vi "VNA_control.vi"() -> ()   [LabVIEW 2013]
uses:
  <vilib>/Utility/file.llb/Write To Spreadsheet File (DBL).vi
  <vilib>/Utility/file.llb/Write To Spreadsheet File (string).vi
panel:
  in  "Save Graph":bool
  in  "Setup":string="DWU868 Measurement"
  in  "RX antenna":string="MAM-DWU868"
  in  "TX antenna":string="BowTie Vertical"
  in  "Polarization":string="Vertical"
  in  "Save Config":bool
  in  "Config Notes":string="6dB attenuation after Amp\n\n360 turn Antenna in center\nTurntabel pot at 100"
  out "10 deg left":bool
  out "Current Angle":i16=-1
  out "Numeric":i32=2991
  in  "Stop Angle":i16=360
  in  "Start Angle":i16
  in  "Save Current Plot Data":bool
  in  "address":i16=26
  in  "bus":i32
  out "Instrument ID":string="HEWLETT PACKARD,8753ES,US39174843,7.74 \n"
  in  "Number of Points":string="401"
  in  "Output Power":string="0"
  in  "IFBW":string="1000"
  in  "Stop Freq. (MHz)":string="2600"
  out "Forced Sweep Time":string="   4.499999948800000E-01\n"
  out "Forced Start Freq.":string="   1.700000000000000E+09\n"
  out "Forced Stop Freq.":string="   2.600000000000000E+09\n"
  out "Forced IFBW":string="   1.000000000000000E+03\n"
  out "Forced Number of Points":string="   4.010000000000000E+02\n"
  out "Forced  Output Power":string="   0.000000000000000E+00\n"
  in  "Start Freq. (MHz)":string="1700"
  out "Freq. Array":dbl[](array[numeric])=[1700000000.0, 1702250000.0, 1704500000.0, 1706750000.0, 1709000000.0, 1711250000.0, 1713500000.0, 1715750000.0, 1718000000.0, 1720250000.0, 1722500000.0, 1724750000.0, 1727000000.0, 1729250000.0, 1731500000.0, 1733750000.0, 1736000000.0, 1738250000.0, 1740500000.0, 1742750000.0, 1745000000.0, 1747250000.0, 1749500000.0, 1751750000.0, 1754000000.0, 1756250000.0, 1758500000.0, 1760750000.0, 1763000000.0, 1765250000.0, 1767500000.0, 1769750000.0, 1772000000.0, 1774250000.0, 1776500000.0, 1778750000.0, 1781000000.0, 1783250000.0, 1785500000.0, 1787750000.0, 1790000000.0, 1792250000.0, 1794500000.0, 1796750000.0, 1799000000.0, 1801250000.0, 1803500000.0, 1805750000.0, 1808000000.0, 1810250000.0, 1812500000.0, 1814750000.0, 1817000000.0, 1819250000.0, 1821500000.0, 1823750000.0, 1826000000.0, 1828250000.0, 1830500000.0, 1832750000.0, 1835000000.0, 1837250000.0, 1839500000.0, 1841750000.0, 1844000000.0, 1846250000.0, 1848500000.0, 1850750000.0, 1853000000.0, 1855250000.0, 1857500000.0, 1859750000.0, 1862000000.0, 1864250000.0, 1866500000.0, 1868750000.0, 1871000000.0, 1873250000.0, 1875500000.0, 1877750000.0, 1880000000.0, 1882250000.0, 1884500000.0, 1886750000.0, 1889000000.0, 1891250000.0, 1893500000.0, 1895750000.0, 1898000000.0, 1900250000.0, 1902500000.0, 1904750000.0, 1907000000.0, 1909250000.0, 1911500000.0, 1913750000.0, 1916000000.0, 1918250000.0, 1920500000.0, 1922750000.0, 1925000000.0, 1927250000.0, 1929500000.0, 1931750000.0, 1934000000.0, 1936250000.0, 1938500000.0, 1940750000.0, 1943000000.0, 1945250000.0, 1947500000.0, 1949750000.0, 1952000000.0, 1954250000.0, 1956500000.0, 1958750000.0, 1961000000.0, 1963250000.0, 1965500000.0, 1967750000.0, 1970000000.0, 1972250000.0, 1974500000.0, 1976750000.0, 1979000000.0, 1981250000.0, 1983500000.0, 1985750000.0, 1988000000.0, 1990250000.0, 1992500000.0, 1994750000.0, 1997000000.0, 1999250000.0, 2001500000.0, 2003750000.0, 2006000000.0, 2008250000.0, 2010500000.0, 2012750000.0, 2015000000.0, 2017250000.0, 2019500000.0, 2021750000.0, 2024000000.0, 2026250000.0, 2028500000.0, 2030750000.0, 2033000000.0, 2035250000.0, 2037500000.0, 2039750000.0, 2042000000.0, 2044250000.0, 2046500000.0, 2048750000.0, 2051000000.0, 2053250000.0, 2055500000.0, 2057750000.0, 2060000000.0, 2062250000.0, 2064500000.0, 2066750000.0, 2069000000.0, 2071250000.0, 2073500000.0, 2075750000.0, 2078000000.0, 2080250000.0, 2082500000.0, 2084750000.0, 2087000000.0, 2089250000.0, 2091500000.0, 2093750000.0, 2096000000.0, 2098250000.0, 2100500000.0, 2102750000.0, 2105000000.0, 2107250000.0, 2109500000.0, 2111750000.0, 2114000000.0, 2116250000.0, 2118500000.0, 2120750000.0, 2123000000.0, 2125250000.0, 2127500000.0, 2129750000.0, 2132000000.0, 2134250000.0, 2136500000.0, 2138750000.0, 2141000000.0, 2143250000.0, 2145500000.0, 2147750000.0, 2150000000.0, 2152250000.0, 2154500000.0, 2156750000.0, 2159000000.0, 2161250000.0, 2163500000.0, 2165750000.0, 2168000000.0, 2170250000.0, 2172500000.0, 2174750000.0, 2177000000.0, 2179250000.0, 2181500000.0, 2183750000.0, 2186000000.0, 2188250000.0, 2190500000.0, 2192750000.0, 2195000000.0, 2197250000.0, 2199500000.0, 2201750000.0, 2204000000.0, 2206250000.0, 2208500000.0, 2210750000.0, 2213000000.0, 2215250000.0, 2217500000.0, 2219750000.0, 2222000000.0, 2224250000.0, 2226500000.0, 2228750000.0, 2231000000.0, 2233250000.0, 2235500000.0, 2237750000.0, 2240000000.0, 2242250000.0, 2244500000.0, 2246750000.0, 2249000000.0, 2251250000.0, 2253500000.0, 2255750000.0, 2258000000.0, 2260250000.0, 2262500000.0, 2264750000.0, 2267000000.0, 2269250000.0, 2271500000.0, 2273750000.0, 2276000000.0, 2278250000.0, 2280500000.0, 2282750000.0, 2285000000.0, 2287250000.0, 2289500000.0, 2291750000.0, 2294000000.0, 2296250000.0, 2298500000.0, 2300750000.0, 2303000000.0, 2305250000.0, 2307500000.0, 2309750000.0, 2312000000.0, 2314250000.0, 2316500000.0, 2318750000.0, 2321000000.0, 2323250000.0, 2325500000.0, 2327750000.0, 2330000000.0, 2332250000.0, 2334500000.0, 2336750000.0, 2339000000.0, 2341250000.0, 2343500000.0, 2345750000.0, 2348000000.0, 2350250000.0, 2352500000.0, 2354750000.0, 2357000000.0, 2359250000.0, 2361500000.0, 2363750000.0, 2366000000.0, 2368250000.0, 2370500000.0, 2372750000.0, 2375000000.0, 2377250000.0, 2379500000.0, 2381750000.0, 2384000000.0, 2386250000.0, 2388500000.0, 2390750000.0, 2393000000.0, 2395250000.0, 2397500000.0, 2399750000.0, 2402000000.0, 2404250000.0, 2406500000.0, 2408750000.0, 2411000000.0, 2413250000.0, 2415500000.0, 2417750000.0, 2420000000.0, 2422250000.0, 2424500000.0, 2426750000.0, 2429000000.0, 2431250000.0, 2433500000.0, 2435750000.0, 2438000000.0, 2440250000.0, 2442500000.0, 2444750000.0, 2447000000.0, 2449250000.0, 2451500000.0, 2453750000.0, 2456000000.0, 2458250000.0, 2460500000.0, 2462750000.0, 2465000000.0, 2467250000.0, 2469500000.0, 2471750000.0, 2474000000.0, 2476250000.0, 2478500000.0, 2480750000.0, 2483000000.0, 2485250000.0, 2487500000.0, 2489750000.0, 2492000000.0, 2494250000.0, 2496500000.0, 2498750000.0, 2501000000.0, 2503250000.0, 2505500000.0, 2507750000.0, 2510000000.0, 2512250000.0, 2514500000.0, 2516750000.0, 2519000000.0, 2521250000.0, 2523500000.0, 2525750000.0, 2528000000.0, 2530250000.0, 2532500000.0, 2534750000.0, 2537000000.0, 2539250000.0, 2541500000.0, 2543750000.0, 2546000000.0, 2548250000.0, 2550500000.0, 2552750000.0, 2555000000.0, 2557250000.0, 2559500000.0, 2561750000.0, 2564000000.0, 2566250000.0, 2568500000.0, 2570750000.0, 2573000000.0, 2575250000.0, 2577500000.0, 2579750000.0, 2582000000.0, 2584250000.0, 2586500000.0, 2588750000.0, 2591000000.0, 2593250000.0, 2595500000.0, 2597750000.0, 2600000000.0]
  in  "Initiate VNA":bool
  in  "Start Turntabel":bool
  out "output array":dbl[](array[numeric])=[-46.14952865404781, -46.232691273557066, -46.2430751503902, -47.25114271797669, -48.120198903692916, -48.730730027922824, -49.09122541047449, -48.90673988745354, -48.544485930725855, -47.554193224998116, -46.87496927167575, -47.323185912630805, -47.33524101209766, -47.700566092891414, -47.92224440903191, -48.31440966542858, -48.44676619037045, -48.369140911799356, -47.9319832767418, -47.79400417552629, -47.695877874655494, -47.27824599163412, -47.543545591805994, -47.85140868427288, -48.01611296880547, -48.53975692801747, -49.98407852530598, -50.26084058142029, -51.97096924166111, -52.47408937498201, -52.98432913841936, -52.98251865389443, -53.182245088383866, -53.73887271810353, -54.03381513974967, -54.53405597057487, -55.14036079577603, -55.09964293760475, -54.37403089032421, -54.509993323127986, -54.132221772847686, -53.93974466854097, -53.872323842183405, -54.5572260055185, -55.082787936170085, -54.76082910636844, -55.36994774177763, -55.04309671548235, -55.05711705014066, -54.743857051015546, -54.95419359130922, -55.453231036245526, -56.620040992534314, -56.933180240449126, -57.98254486940575, -58.47116123008044, -57.63144943704836, -56.354612757402826, -56.33945467985886, -55.55041492411028, -55.13498792296701, -54.98928915550141, -53.54147323007345, -53.0866987847333, -51.49720736907496, -50.65872377331299, -49.429444691265175, -49.00066533585979, -49.18236382208785, -48.7346651816435, -48.6428733454471, -49.0369511760136, -49.647405916877204, -49.91495131123127, -50.73332378781956, -51.146640766658365, -53.274167053780715, -53.07556548774521, -54.967399293132374, -54.91558848425554, -54.981529686395916, -53.81281146841167, -52.721668856936496, -52.29174907211479, -51.30755297551491, -51.555344613413695, -51.49437195127626, -50.859642725917915, -50.47279848060345, -50.16547905504841, -49.515991937660516, -48.996309364354886, -48.5516751819824, -49.024107657150886, -49.91174729634915, -50.07206023503437, -50.354983564457726, -50.392253363720755, -50.47806698290641, -51.51467197522007, -51.351231626270355, -51.69316044997287, -53.26430703058692, -54.35675089190596, -54.85802150691952, -54.704993318181884, -55.76726541464235, -54.59961731237464, -53.30318902070684, -52.94609349489569, -52.022734676258466, -52.11828429214016, -51.638575770160706, -51.01379988123214, -50.81589628452204, -50.87648726039296, -50.574567626726726, -50.64041926852853, -51.23049863941315, -52.77518876786951, -54.565252786618956, -55.67713448969707, -54.97657805901591, -55.08819292455469, -53.636596755806, -52.06216902185375, -51.753902007901964, -51.362001769216164, -51.22852523767171, -50.859218499788064, -51.50091639754157, -52.16908806766697, -52.20245674039589, -52.78518708052982, -52.48479007561359, -52.32892136658103, -52.26852911390827, -52.13380162088395, -51.77905530163895, -52.735823457055815, -53.81481636754703, -54.75341742214041, -54.940658392596305, -56.054572522496755, -58.47243572834671, -57.76124622271905, -57.058175267930274, -56.269775356868635, -55.045786149128375, -53.446627798069, -52.86588443898755, -53.08744436022421, -53.11735575591441, -53.765960092523606, -54.04943344923838, -53.86246333075452, -53.63391540269025, -52.562326184283066, -52.18242551834151, -51.662691717319504, -52.048603771022385, -51.96139467528154, -52.349486330100284, -53.071788933659725, -53.915943306995786, -55.505890401255925, -56.576757954112225, -57.4142046921861, -60.01099137822906, -58.18265447419201, -58.46272582985546, -56.72814383384765, -56.138856824351464, -54.92303353601231, -54.13069037615369, -54.041884744102695, -53.52403819998679, -52.75135112760272, -52.664887440409785, -51.46976083524018, -51.585128029137564, -51.31789520890483, -50.968888605370694, -50.84010994573585, -51.375048830498145, -51.4022248032098, -51.79429768890644, -52.64804024181253, -53.95089200145986, -55.64999686317979, -56.527693517294004, -57.93929882997876, -58.18334879548402, -56.74120095178944, -56.32073895503707, -55.095781520608696, -54.640016588348104, -54.16375042634547, -53.54090662420656, -53.155620894520524, -52.89394954756738, -52.14525498371656, -52.14636786851274, -52.25143622782487, -52.823523428578156, -54.17398555442098, -54.36688985412034, -54.34227843986237, -54.58314609059877, -54.57723755565346, -54.105672986039856, -54.889370038295866, -55.98966342846481, -57.24096049907829, -59.98627732389639, -58.50017548457405, -58.501426766481714, -56.23661821314542, -54.95043675718922, -54.127780510113, -53.450576979909385, -53.63090794550815, -53.928380762141984, -54.13683658276507, -54.540962001289415, -54.86955512548106, -55.34394924932282, -55.15981874534231, -55.28640089518934, -55.46842364266997, -55.81223725249389, -56.395570583459175, -56.29175492961587, -56.83404549292931, -57.8393031277243, -57.64316593133805, -57.29374553728293, -57.00104583682321, -57.57344727121647, -58.09325416171514, -57.57483582826591, -55.78214269066137, -55.261525588080794, -54.02783172166294, -53.57537740207282, -53.52052550346449, -53.68735889131014, -55.18092983656392, -56.34549876165538, -55.918397497849746, -55.35119850754077, -55.94772721336473, -55.82941229807342, -55.20278579555211, -54.948624944647776, -55.96472293595988, -56.93216605743473, -56.62091714768949, -56.344134807314, -56.87589189638767, -58.07588784043862, -56.61746447511564, -57.37793393626014, -56.544796647017954, -56.84017188827894, -55.6548966978255, -54.893537730518986, -53.959397461583514, -55.03887939804265, -54.965845039381584, -54.31395807000967, -54.358759341780285, -55.33356078933967, -56.225359077155275, -55.65103376805243, -55.26348670787047, -55.467908232117686, -55.16848650302911, -54.88731484218719, -54.9758391979146, -55.64412397666068, -56.96934756557026, -57.65955600340944, -55.916224294186776, -55.612167236283405, -55.96308576364933, -56.05231864509027, -55.25347599171945, -55.304583268840524, -55.69757297967533, -56.195809454262246, -54.82790811670832, -54.31342240066522, -54.6145369456925, -54.4531761464751, -53.96187197225166, -53.78090109665749, -53.85330013355278, -54.31466736083655, -54.5671580183431, -54.40724045187317, -55.490000620727315, -56.18920098061764, -57.25904466242302, -58.243628500935955, -58.79003501603385, -60.14505058874654, -60.14278073191541, -60.07809070689417, -57.809595741609165, -58.25229962043673, -58.33514185743652, -58.27537699051207, -57.982458817507876, -57.32506348305857, -56.66224565603442, -55.51869934148086, -54.691925020045645, -54.10692375027259, -54.900046526270444, -54.933692151675906, -56.019032428599985, -55.34456759853007, -55.953658267597184, -56.3791344707824, -56.26438578443476, -56.93526534183916, -57.33423251579217, -58.07822806088768, -58.76243251365143, -58.67133015427089, -58.28982113165295, -58.95225990994228, -58.67126209522736, -57.89987614108138, -57.72620629786993, -57.62425975451958, -56.97306879778283, -57.70848962384082, -57.357219867042076, -57.42349439048927, -57.64482666750731, -58.34784235225299, -57.311726932236496, -57.09929950493894, -57.04169634219369, -57.9138740414414, -57.726322625896415, -57.43839965210705, -57.30879814697985, -57.40503608346495, -56.91037950988086, -57.31970259346343, -58.5831639851512, -59.57149175879184, -60.71303717626585, -61.48630455672968, -61.31227523849908, -61.539120672976686, -60.982442738400195, -60.83008160295606, -60.3810650516995, -60.11182688482912, -60.14622384911674, -59.536412725623045, -58.466165432555556, -58.211492553458406, -57.70695649674601, -56.87189462723518, -56.347512153121706, -56.03399358565113, -56.42318400860642, -57.28869218804995, -58.22846603399611, -58.63279363791775, -58.59667261259264, -59.005226463047904, -58.815012450001504, -58.33561529066227, -58.02667764914552, -58.33733261314406, -58.62425246039699, -58.040265154895366, -56.91046547462501, -57.706983087948785, -59.010485928120886, -58.97101422590738, -59.0853283186, -59.39769414728251, -60.25211579991711, -59.7957969175217, -59.46973747494233, -58.84867051731946, -58.732266964976205, -58.63718591494741, -58.359292232606315, -58.15315438077847, -58.86195256988518, -59.5661822007773, -60.74784745212166, -60.516354440305406]
  in  "Capture Data":bool
  in  "stop":bool
  out "XY Graph":cluster{"Freq. Array":dbl[], dbl[]}(graph)
  in  "Serial Port":refnum<visa-resource-name>="ASRL4::INSTR"
  out "DCD":bool
  # "SMP VNA: 26"
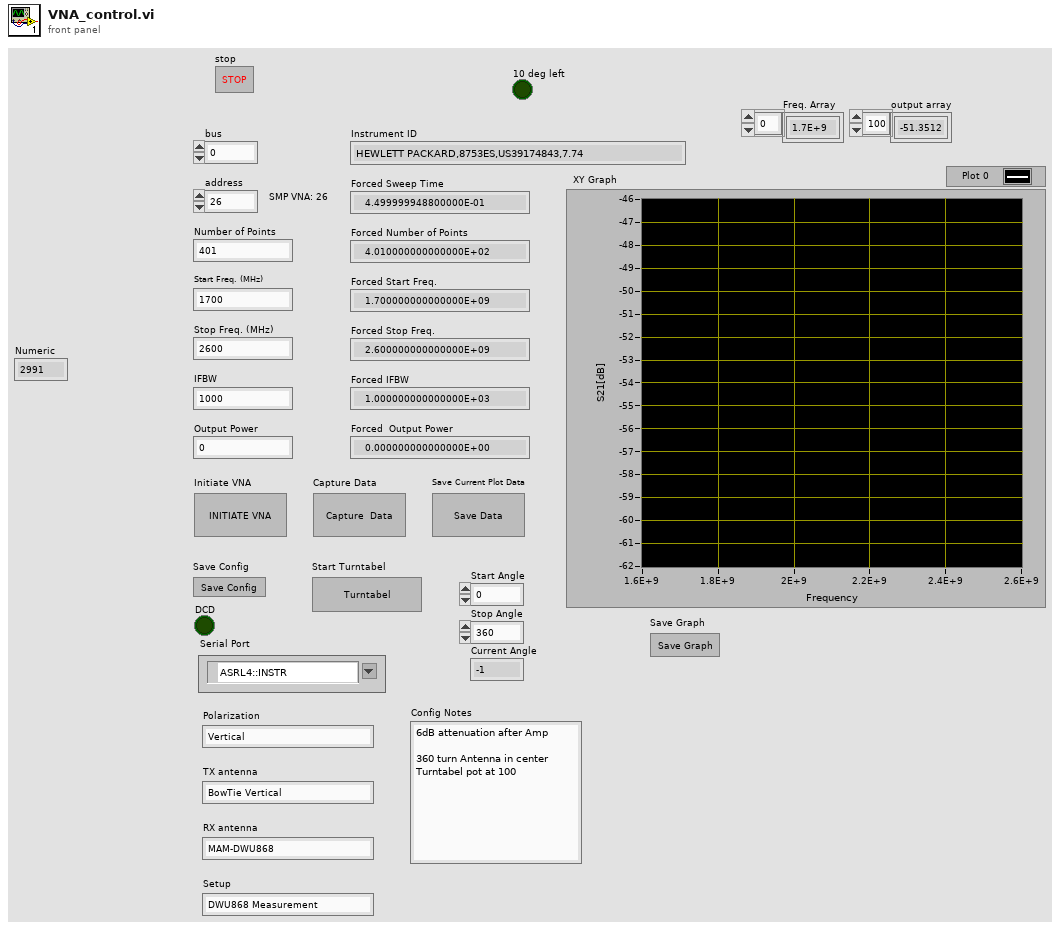
[diagram p1: front panel]
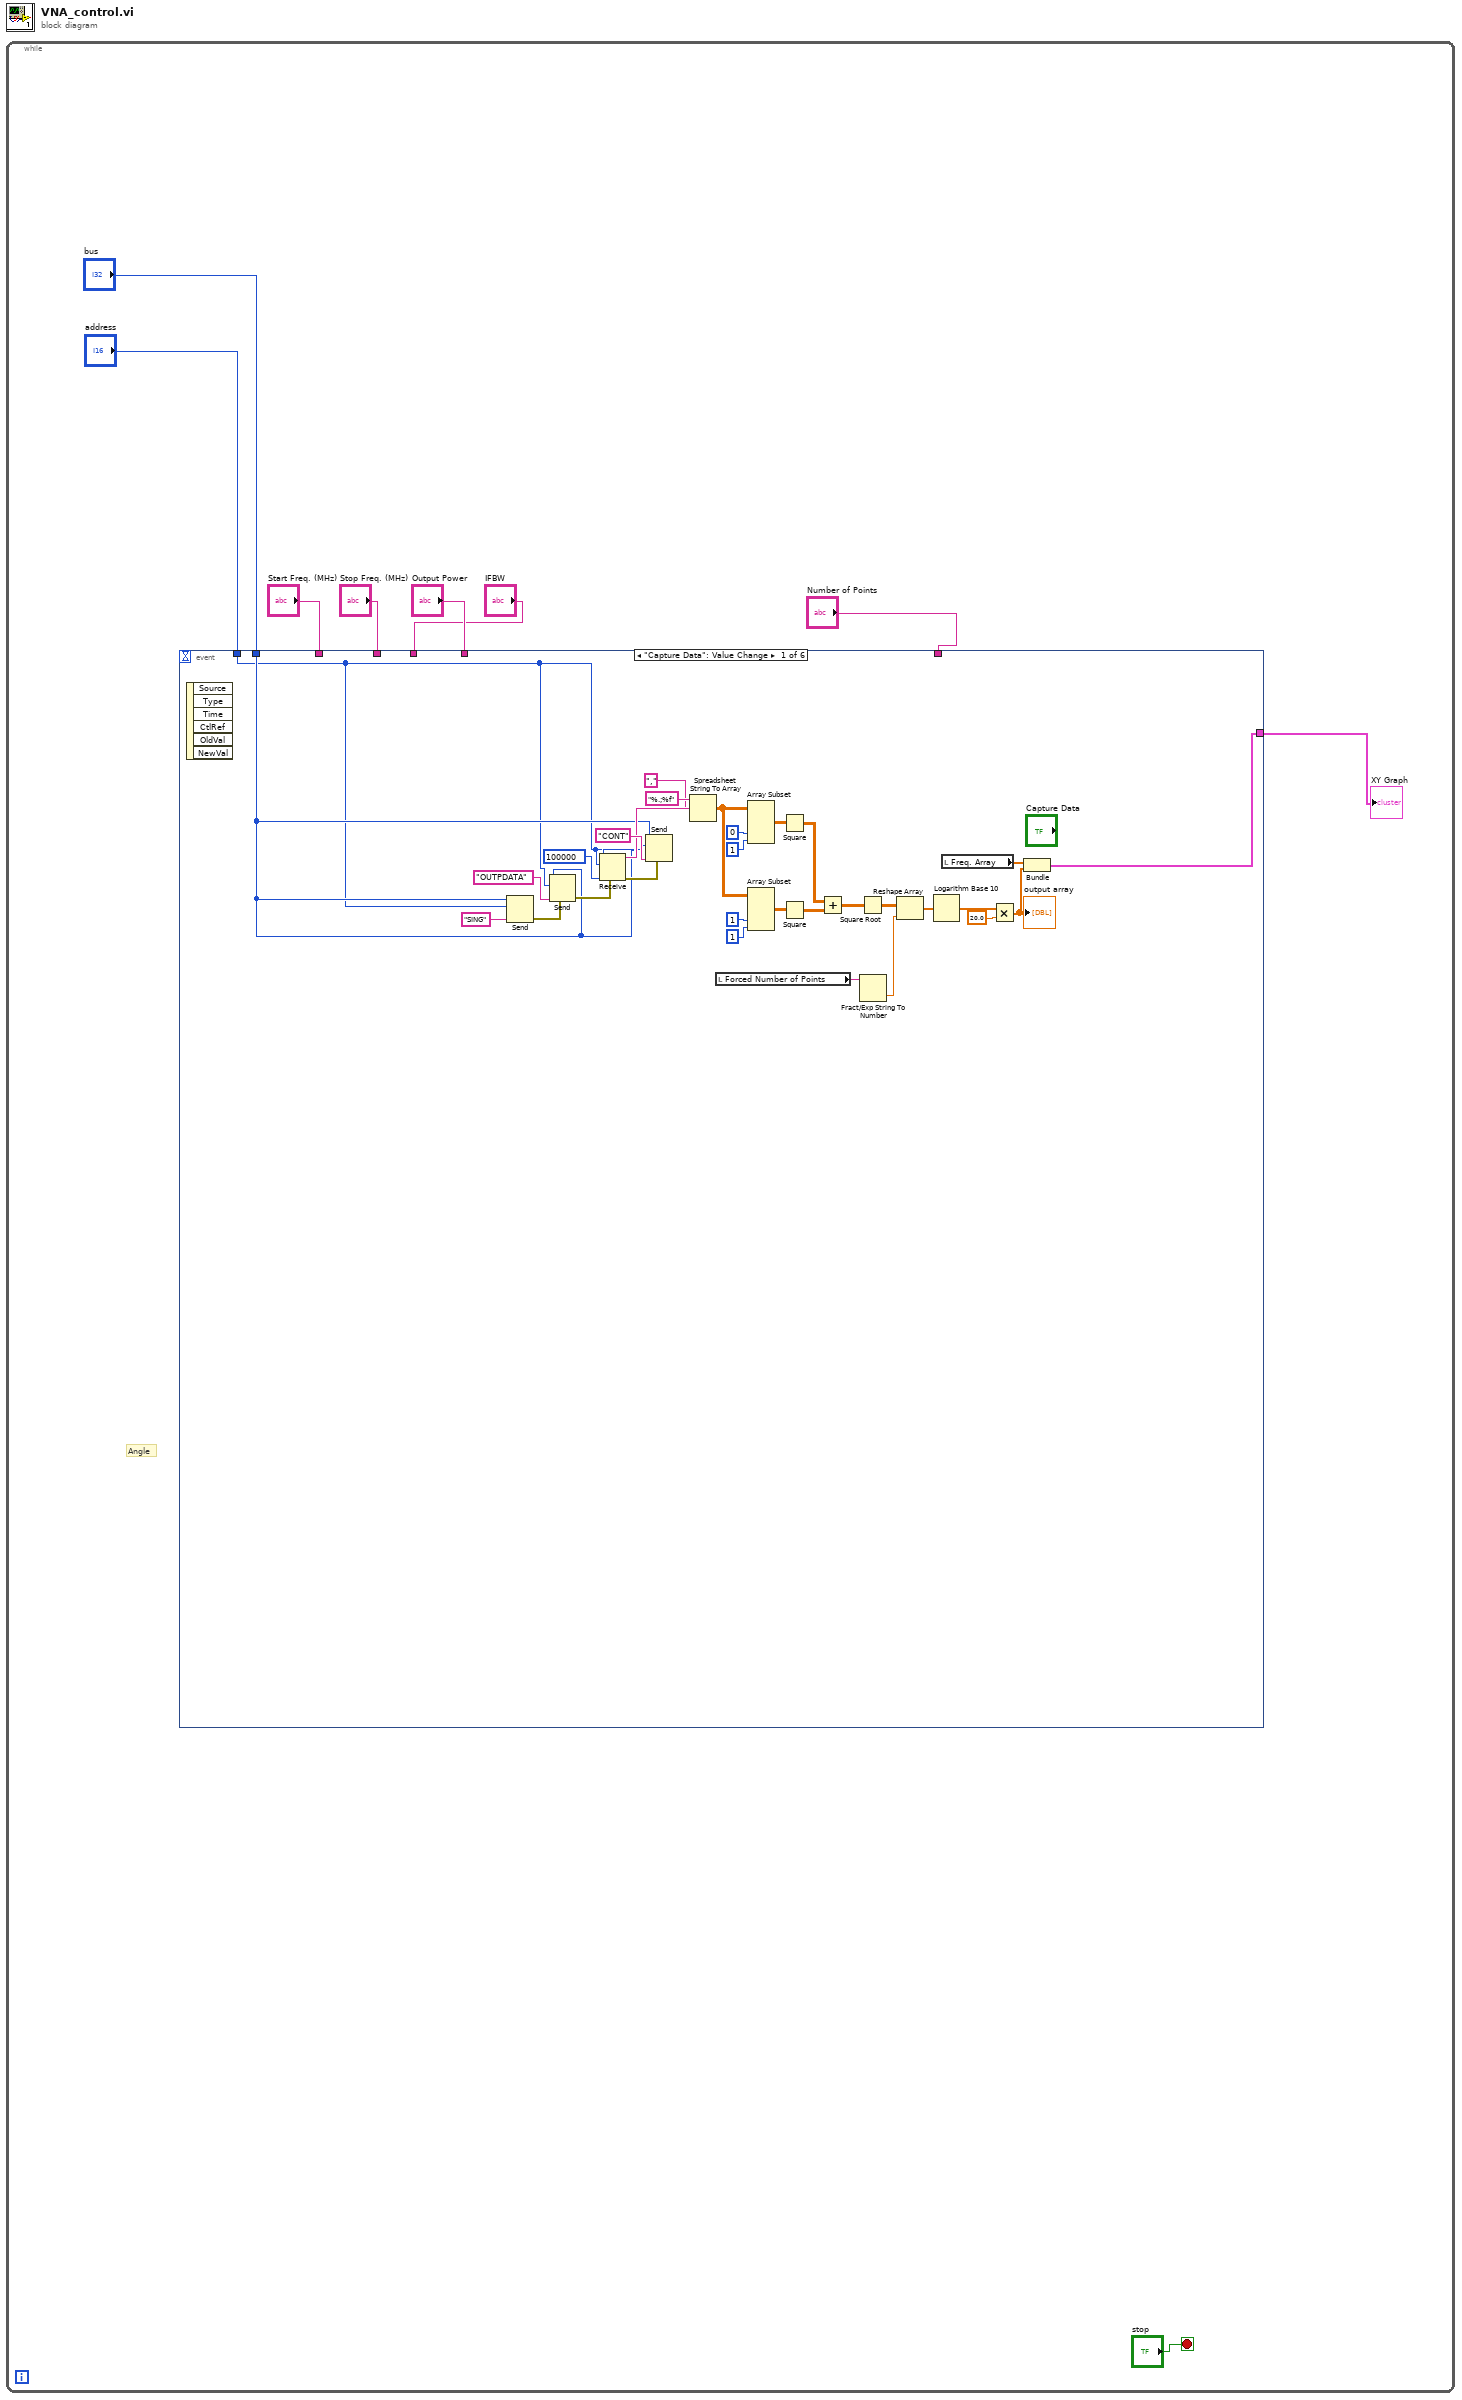
[diagram p0: block diagram]
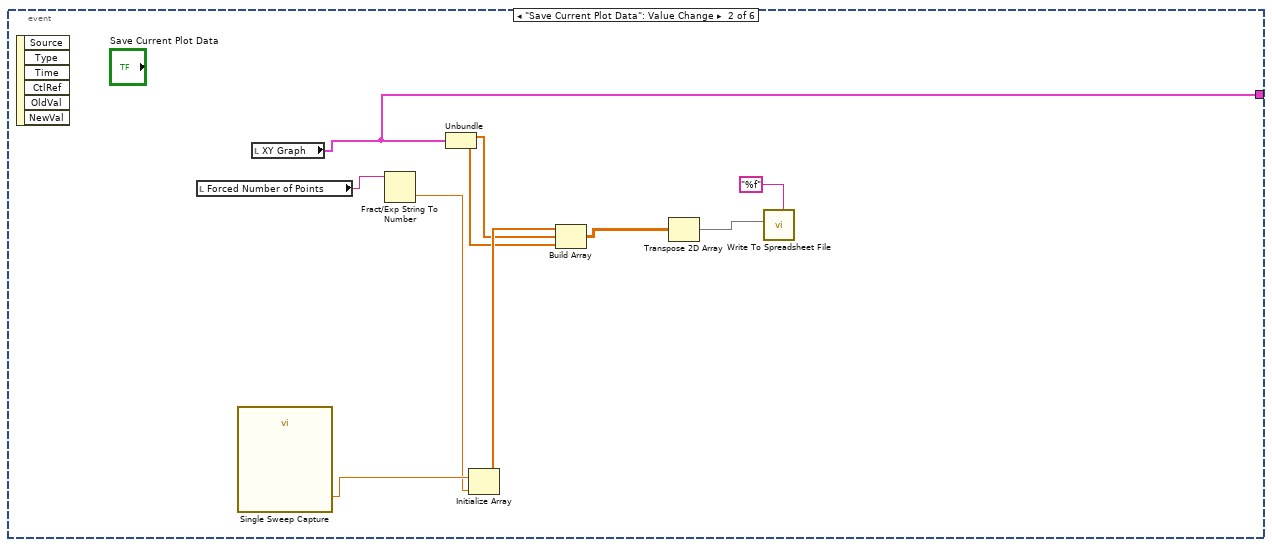
[diagram p2: hidden frame]
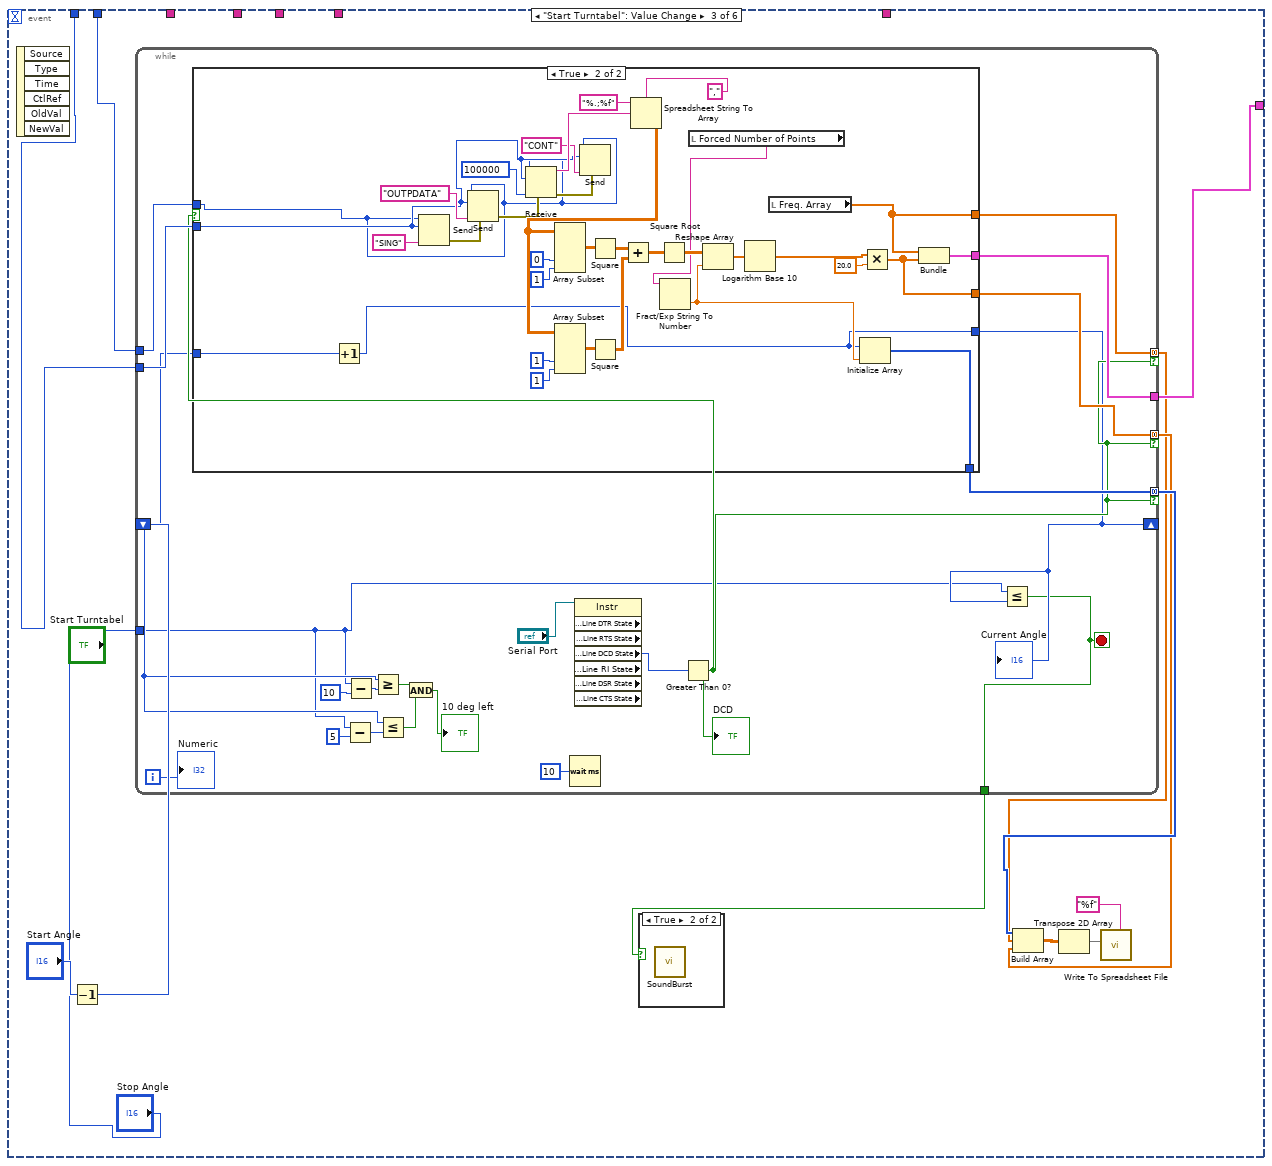
[diagram p3: hidden frame]
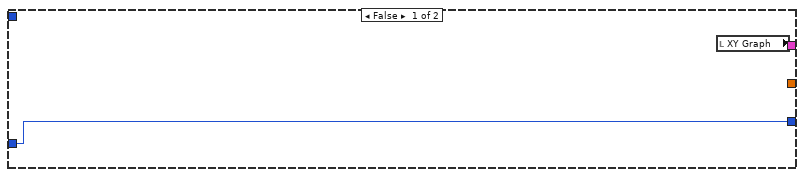
[diagram p5: hidden frame]
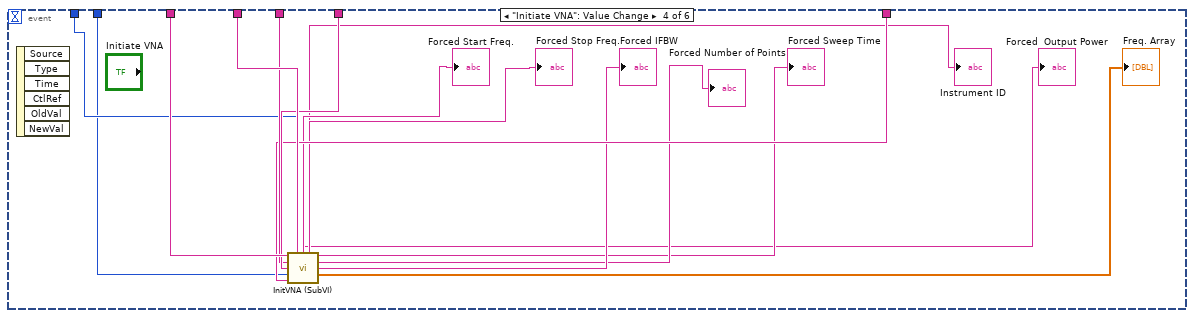
[diagram p6: hidden frame]
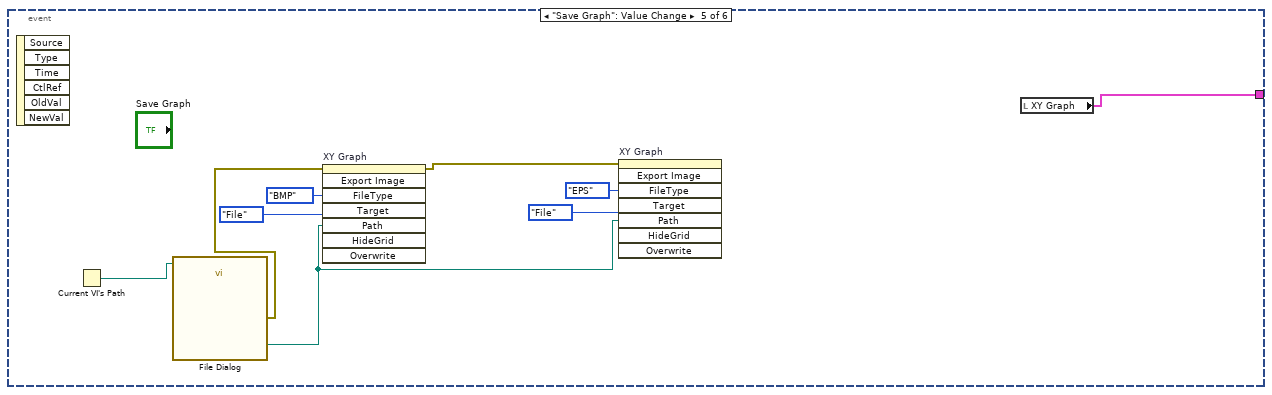
[diagram p7: hidden frame]
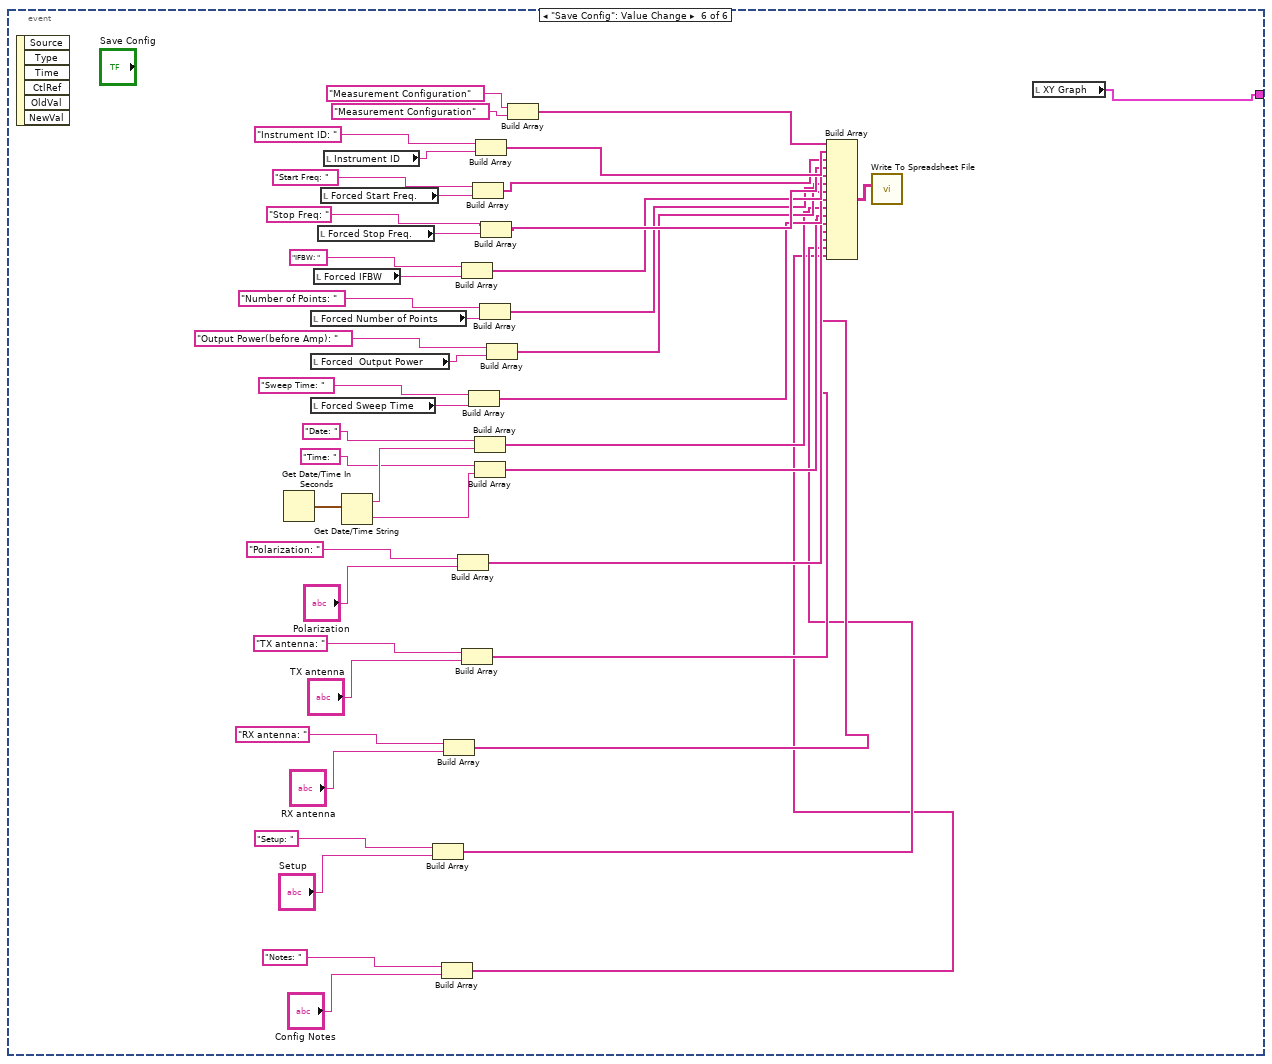
[diagram p8: hidden frame]
diagram:
  n1 = while {
    stop <- "stop" stop-if-true
    # "Angle"
    n2 = event shown="[0] \"Capture Data\": Value Change" {
      selector: _ -> [_ _ _ _ _ _]
      dyn-events: _ -> [_ _ _ _ _ _]
      timeout: _ -> [_ _ _ _ _ _]
      tunnel: "bus" -> [w20 _ w61 w130 _ _]
      tunnel: "address" -> [w19 _ w62 w131 _ _]
      tunnel: "Number of Points" -> [_ _ _ w132 _ _]
      tunnel: [w12 w42 w60 _ w137 w146] -> w5
      tunnel: "Start Freq. (MHz)" -> [_ _ _ w136 _ _]
      tunnel: "Stop Freq. (MHz)" -> [_ _ _ w135 _ _]
      tunnel: "Output Power" -> [_ _ _ w134 _ _]
      tunnel: "IFBW" -> [_ _ _ w133 _ _]
      event "Capture Data": Value Change {
        n3 = event-data() -> ()  [unwired: 1 in, 6 out]
        n4 = Send(0:w20, 2:w19, 5:"SING" ("data string")) -> (8:w38:errorcluster)  [unwired: 2 in, 2 out]
        n5 = Send(0:w20, 2:w19, 4:w38, 5:"OUTPDATA" ("data string")) -> (8:w37:errorcluster)  [unwired: 1 in, 2 out]
        n6 = Receive(4:w37, 6:100000 ("byte count"), 8:w19, 9:w20) -> (0:w36:errorcluster, 3:w33:string)  [unwired: 1 in, 2 out]
        n7 = Send(0:w20, 2:w19, 4:w36, 5:"CONT" ("data string")) -> ()  [unwired: 1 in, 3 out]
        n8 = Spreadsheet String To Array(delimiter (Tab)=",", format string="%.;%f", spreadsheet string=w33) -> (array=w30:dbl[][])  [unwired: 1 in]
        n9 = local read "Forced Number of Points"() -> (w10:string)
        n10 = Array Subset(array=w30, index (col)=0 ("index"), length (col)=1 ("length")) -> (w25:dbl[][])  [unwired: 2 in]
        n11 = Array Subset(array=w30, index (col)=1 ("index"), length (col)=1 ("length")) -> (w24:dbl[][])  [unwired: 2 in]
        n12 = Square(x=w25) -> (x^2=w22:dbl[][])
        n13 = Square(x=w24) -> (x^2=w23:dbl[][])
        n14 = Add(x=w22, y=w23) -> (x+y=w21:dbl[][])
        n15 = Square Root(x=w21) -> (sqrt(x)=w18:dbl[][])
        n16 = Fract/Exp String To Number(string=w10) -> (number=w17:dbl)  [unwired: 3 in, 1 out]
        n17 = Reshape Array(w18, w17) -> (w16:dbl[])
        n18 = Logarithm Base 10(1:w16) -> (0:w13:dbl[])
        n19 = local read "Freq. Array"() -> (w11:dbl[])
        n20 = Multiply(x=w13, y=20.0) -> (x*y=w15:dbl[])
        "output array" <- w15
        n21 = Bundle("Freq. Array"=w11, w15) -> (w12:cluster{"Freq. Array":dbl[], dbl[]})  [unwired: 1 in]
      }
      event "Save Current Plot Data": Value Change {
        n22 = event-data() -> ()  [unwired: 1 in, 6 out]
        n23 = local read "Forced Number of Points"() -> (w48:string)
        n24 = call "Single Sweep Capture"() -> ("Angle"=w49:dbl)  [unwired: 17 in, 2 out]
        n25 = local read "XY Graph"() -> (w42:cluster{"Freq. Array":dbl[], dbl[]})
        n26 = Fract/Exp String To Number(string=w48) -> (number=w47:dbl)  [unwired: 3 in, 1 out]
        n27 = Unbundle(w42) -> ("Freq. Array"=w45:dbl[], w44:dbl[])
        n28 = Initialize Array(w49, w47) -> (w46:dbl[])
        n29 = Build Array(w46, w45, w44) -> (w43:dbl[][])
        n30 = Transpose 2D Array(2D array=w43) -> (transposed array=w50:dbl[][])
        n31 = call-poly <vilib>:"Write To Spreadsheet File.vi"("format (%.3f)"="%f", "2D data"=w50) -> ()  [unwired: 6 in, 1 out]
      }
      event "Start Turntabel": Value Change {
        n32 = event-data() -> ()  [unwired: 1 in, 6 out]
        n33 = Decrement(x="Start Angle") -> (x-1=w56:i16)
        n34 = while {
          tunnel: w62 -> [w82]
          tunnel: w61 -> [w81]
          tunnel: [w79] -> w60
          shift-right: [w74] -> _
          shift-left: w56 -> [w66]
          tunnel: [w78] -> w58 mode=concatenating if=w76
          tunnel: [w77] -> w59 mode=concatenating if=w76
          tunnel: [w80] -> w57 mode=concatenating if=w76
          tunnel: "Stop Angle" -> [w65]
          tunnel: [w64] -> w52
          i -> [w73]
          stop <- w64 stop-if-true
          n35 = Subtract(x=w65, y=i16 5) -> (x-y=w70:i16)
          n36 = Subtract(x=w65, y=i16 10) -> (x-y=w72:i16)
          n37 = Greater Or Equal?(x=w66, y=w72) -> (x >= y?=w69:bool)
          n38 = Less Or Equal?(x=w66, y=w70) -> (x <= y?=w68:bool)
          n39 = And(x=w69, y=w68) -> (x .and. y?=→"10 deg left":bool)
          n40 = Wait (ms)(milliseconds to wait=u32 10) -> ()  [unwired: 1 out]
          n41 = property class="Instr" props=["Serial Settings:Modem Line Settings:Line DTR State", "Serial Settings:Modem Line Settings:Line RTS State", "Serial Settings:Modem Line Settings:Line DCD State", "Serial Settings:Modem Line Settings:Line RI State", "Serial Settings:Modem Line Settings:Line DSR State", "Serial Settings:Modem Line Settings:Line CTS State"](reference="Serial Port") -> ("Serial Settings:Modem Line Settings:Line DCD State"=w84:i16)  [unwired: 1 in, 7 out]
          n42 = Greater Than 0?(x=w84) -> (x > 0?=w76:bool)
          "DCD" <- w76
          n43 = case shown="True" w76 {
            tunnel: w66 -> [w87 w97]
            tunnel: w82 -> [_ w96]
            tunnel: w81 -> [_ w95]
            tunnel: [_ w94] -> w80
            tunnel: [w86 w93] -> w79
            tunnel: [_ w92] -> w78
            tunnel: [_ w91] -> w77
            tunnel: [w87 w90] -> w74
            frame False {
              n44 = local read "XY Graph"() -> (w86:cluster{"Freq. Array":dbl[], dbl[]})
            }
            frame True {
              n45 = Increment(x=w97) -> (x+1=w90:i16)
              n46 = Send(0:w95, 2:w96, 5:"SING" ("data string")) -> (8:w100:errorcluster)  [unwired: 2 in, 2 out]
              n47 = Send(0:w95, 2:w96, 4:w100, 5:"OUTPDATA" ("data string")) -> (8:w101:errorcluster)  [unwired: 1 in, 2 out]
              n48 = Receive(4:w101, 6:100000 ("byte count"), 8:w96, 9:w95) -> (0:w102:errorcluster, 3:w105:string)  [unwired: 1 in, 2 out]
              n49 = Send(0:w95, 2:w96, 4:w102, 5:"CONT" ("data string")) -> ()  [unwired: 1 in, 3 out]
              n50 = Spreadsheet String To Array(delimiter (Tab)=",", format string="%.;%f", spreadsheet string=w105) -> (array=w107:dbl[][])  [unwired: 1 in]
              n51 = Array Subset(array=w107, index (col)=0 ("index"), length (col)=1 ("length")) -> (w112:dbl[][])  [unwired: 2 in]
              n52 = Array Subset(array=w107, index (col)=1 ("index"), length (col)=1 ("length")) -> (w113:dbl[][])  [unwired: 2 in]
              n53 = Square(x=w112) -> (x^2=w115:dbl[][])
              n54 = Square(x=w113) -> (x^2=w114:dbl[][])
              n55 = Add(x=w115, y=w114) -> (x+y=w116:dbl[][])
              n56 = Square Root(x=w116) -> (sqrt(x)=w117:dbl[][])
              n57 = local read "Forced Number of Points"() -> (w89:string)
              n58 = Fract/Exp String To Number(string=w89) -> (number=w121:dbl)  [unwired: 3 in, 1 out]
              n59 = Reshape Array(w117, w121) -> (w118:dbl[])
              n60 = Logarithm Base 10(1:w118) -> (0:w120:dbl[])
              n61 = local read "Freq. Array"() -> (w94:dbl[])
              n62 = Initialize Array(w90, w121) -> (w91:i16[])
              n63 = Multiply(x=w120, y=20.0) -> (x*y=w92:dbl[])
              n64 = Bundle("Freq. Array"=w94, w92) -> (w93:cluster{"Freq. Array":dbl[], dbl[]})  [unwired: 1 in]
            }
          }
          "Current Angle" <- w74
          n65 = Less Or Equal?(x=w65, y=w74) -> (x <= y?=w64:bool)
          "Numeric" <- w73
        }
        n66 = case shown="True" w52 {
          frame False {
          }
          frame True {
            n67 = call "SoundBurst.vi"() -> ()  [unwired: 12 in]
          }
        }
        n68 = Build Array(w59, w57, w58) -> (w53:dbl[][])
        n69 = Transpose 2D Array(2D array=w53) -> (transposed array=w63:dbl[][])
        n70 = call-poly <vilib>:"Write To Spreadsheet File.vi"("format (%.3f)"="%f", "2D data"=w63) -> ()  [unwired: 6 in, 1 out]
      }
      event "Initiate VNA": Value Change {
        n71 = event-data() -> ()  [unwired: 1 in, 6 out]
        n72 = call "InitVNA (SubVI).vi"("Start Freq. (MHz)"=w136, "Stop Freq. (MHz)"=w135, "IFBW"=w133, "Output Power"=w134, "bus"=w130, "Number of Points"=w132, "address"=w131) -> ("Forced  Output Power"=→"Forced  Output Power":string, "Instrument ID"=→"Instrument ID":string, "Forced Sweep Time"=→"Forced Sweep Time":string, "Forced Number of Points"=→"Forced Number of Points":string, "Forced IFBW"=→"Forced IFBW":string, "Freq. Array"=→"Freq. Array":dbl[], "Forced Start Freq."=→"Forced Start Freq.":string, "Forced Stop Freq."=→"Forced Stop Freq.":string)  [unwired: 1 out]
      }
      event "Save Graph": Value Change {
        n73 = event-data() -> ()  [unwired: 1 in, 6 out]
        n74 = Current VI's Path() -> (path=w139:path)
        n75 = call "File Dialog"("start path"=w139) -> ("selected path"=w140:path, "error out"=w138:errorcluster)  [unwired: 11 in, 2 out]
        n76 = invoke on="XY Graph" class="XYGraph (strict)" method="Export Image"(error in=w138, "FileType"=enum32{"BMP", "EPS", "EMF", "PICT"}."BMP" ("File Type"), "Target"=enum32{"File", "Clipboard"}."File", "Path"=w140) -> (error out=w143:errorcluster)  [unwired: 4 in, 7 out]
        n77 = invoke on="XY Graph" class="XYGraph (strict)" method="Export Image"(error in=w143, "FileType"=enum32{"BMP", "EPS", "EMF", "PICT"}."EPS" ("File Type"), "Target"=enum32{"File", "Clipboard"}."File", "Path"=w140) -> ()  [unwired: 4 in, 8 out]
        n78 = local read "XY Graph"() -> (w137:cluster{"Freq. Array":dbl[], dbl[]})
      }
      event "Save Config": Value Change {
        n79 = event-data() -> ()  [unwired: 1 in, 6 out]
        n80 = Get Date/Time In Seconds() -> (seconds since 1Jan1904=w166:timestamp)
        n81 = local read "Forced Number of Points"() -> (w183:string)
        n82 = local read "Forced  Output Power"() -> (w182:string)
        n83 = local read "Forced Sweep Time"() -> (w181:string)
        n84 = local read "Forced IFBW"() -> (w184:string)
        n85 = local read "Forced Stop Freq."() -> (w178:string)
        n86 = local read "Forced Start Freq."() -> (w185:string)
        n87 = local read "Instrument ID"() -> (w186:string)
        n88 = Get Date/Time String(seconds (now)=w166) -> (date string=w165:string, time string=w164:string)  [unwired: 2 in]
        n89 = Build Array("Setup: " ("string"), "Setup") -> (w148:string[])
        n90 = Build Array("Notes: " ("string"), "Config Notes") -> (w147:string[])
        n91 = Build Array("RX antenna: " ("string"), "RX antenna") -> (w149:string[])
        n92 = Build Array("Polarization: " ("string"), "Polarization") -> (w151:string[])
        n93 = Build Array("IFBW: " ("string"), w184) -> (w174:string[])
        n94 = Build Array("TX antenna: " ("string"), "TX antenna") -> (w150:string[])
        n95 = Build Array("Sweep Time: " ("string"), w181) -> (w171:string[])
        n96 = Build Array("Start Freq: " ("string"), w185) -> (w176:string[])
        n97 = Build Array("Date: " ("string"), w165) -> (w161:string[])
        n98 = Build Array("Time: " ("string"), w164) -> (w160:string[])
        n99 = Build Array("Instrument ID: " ("string"), w186) -> (w177:string[])
        n100 = Build Array("Number of Points: " ("string"), w183) -> (w173:string[])
        n101 = Build Array("Stop Freq: " ("string"), w178) -> (w175:string[])
        n102 = Build Array("Output Power(before Amp): " ("string"), w182) -> (w172:string[])
        n103 = Build Array("Measurement Configuration", "Measurement Configuration") -> (w168:string[])
        n104 = Build Array(w168, w177, w176, w175, w174, w173, w172, w171, w161, w160, w151, w150, w149, w148, w147) -> (w167:string[][])
        n105 = call-poly <vilib>:"Write To Spreadsheet File.vi"("2D data"=w167) -> ()  [unwired: 7 in, 1 out]
        n106 = local read "XY Graph"() -> (w146:cluster{"Freq. Array":dbl[], dbl[]})
      }
    }
    "XY Graph" <- w5
  }
